vi "Inst.Xeryon-Rotator.GetAllData.vi"(8 "error in (no error)":errorcluster, 11 "Inst.Xeryon-Rotator in":refnum<class "Inst.Xeryon-Rotator.lvclass">) -> (0 "error out":errorcluster, 2 "Data out":variant, 3 "Inst.Xeryon-Rotator out":refnum<class "Inst.Xeryon-Rotator.lvclass">)   [LabVIEW 2019, in "Inst.Xeryon-Rotator.lvclass"]
uses:
  Inst.Xeryon-Rotator.lvclass
  Typedefs/Inst.Xeryon-Rotator.getAll--Cluster.ctl
  Inst.Xeryon-Rotator.lvclass/Inst.Xeryon-Rotator.ctl
  Controller.LV/Controller.LV.lvclass
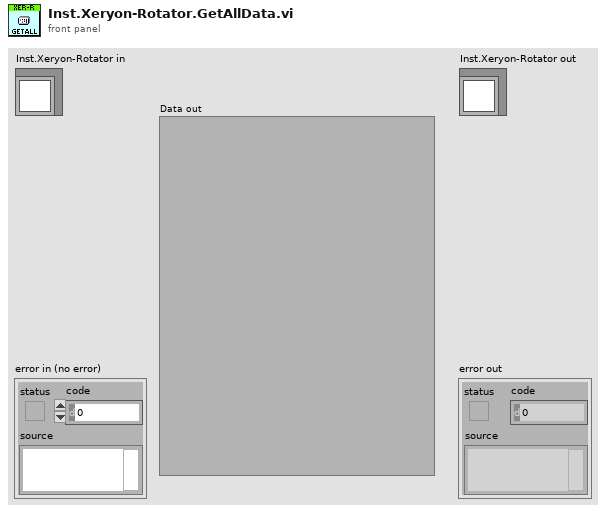
[diagram p1: front panel]
types:
  T1 = typedef "Inst.Xeryon-Rotator.lvclass/Inst.Xeryon-Rotator.getAll--Cluster.ctl" = cluster{"Encoder position [selected units]":dbl, "Desired Position [selected units]":dbl, "Status":string, "SRNO":dbl, "SOFT":dbl, "STAT":dbl, "FREQ":dbl, "OFRQ":dbl, "CURR":dbl, "SYNC":dbl, "Encoder Position [enc. units]":dbl, "Desired Position [enc. units]":dbl, "TIME":dbl, "Index Found":bool, "Left Limit":bool, "Right Limit":bool, "Position Reached":bool}
  T2 = cluster{"SRNO":dbl, "SOFT":dbl, "STAT":dbl, "FREQ":dbl, "OFRQ":dbl, "CURR":dbl, "SYNC":dbl, "Encoder Position [enc. units]":dbl, "Desired Position [enc. units]":dbl, "TIME":dbl}
  T3 = cluster{"Index Found":bool, "Left Limit":bool, "Right Limit":bool, "Position Reached":bool}
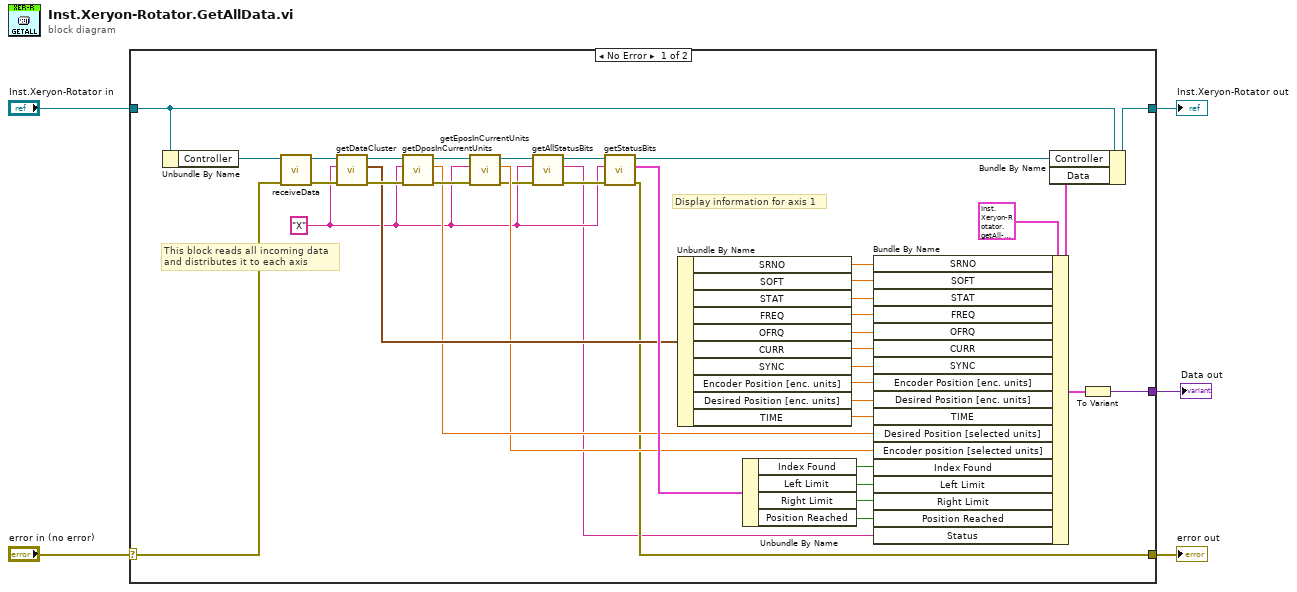
[diagram p0: block diagram]
diagram:
  n1 = case shown="No Error" "error in (no error)" {
    selector: "error in (no error)" -> [w34 w46]
    tunnel: [w13 w46] -> w4
    tunnel: [w44 w45] -> w2
    tunnel: "Inst.Xeryon-Rotator in" -> [w43 w45]
    tunnel: [w42 _] -> w1
    frame No Error {
      w7 = "X" ("Axis Letter")
      # "Display information for axis 1"
      # "This block reads all incoming data\nand distributes it to each axis"
      n2 = Unbundle By Name(w43) -> ("Controller"=w32:refnum<class "Controller.LV.lvclass">)
      n3 = call-dynamic "receiveData.vi"("error in (no error)"=w34, "Controller in"=w32) -> ("error out"=w37:errorcluster, "Controller out"=w36:refnum<class "Controller.LV.lvclass">)  [unwired: 8 in]
      n4 = call-dynamic "getDataCluster.vi"("error in (no error)"=w37, "Axis Letter"=w7, "Controller in"=w36) -> ("error out"=w40:errorcluster, "Information"=w16:T2, "Controller out"=w38:refnum<class "Controller.LV.lvclass">)  [unwired: 6 in]
      n5 = call-dynamic "getDposInCurrentUnits.vi"("error in (no error)"=w40, "Axis Letter"=w7, "Controller in"=w38) -> ("error out"=w41:errorcluster, "DPOS In Current Units"=w15:dbl, "Controller out"=w39:refnum<class "Controller.LV.lvclass">)  [unwired: 6 in]
      n6 = call-dynamic "getEposInCurrentUnits.vi"("error in (no error)"=w41, "Axis Letter"=w7, "Controller in"=w39) -> ("error out"=w10:errorcluster, "EPOS In Current Units"=w14:dbl, "Controller out"=w11:refnum<class "Controller.LV.lvclass">)  [unwired: 6 in]
      n7 = call "getAllStatusBits.vi"("error in (no error)"=w10, "Axis Letter"=w7, "Controller.LV in"=w11) -> ("error out"=w8:errorcluster, "STAT"=w6:string, "Controller.LV out"=w9:refnum<class "Controller.LV.lvclass">)  [unwired: 6 in]
      n8 = call-dynamic "getStatusBits.vi"("error in (no error)"=w8, "Axis Letter"=w7, "Controller in"=w9) -> ("error out"=w13:errorcluster, "StatusBits"=w17:T3, "Controller out"=w35:refnum<class "Controller.LV.lvclass">)  [unwired: 6 in]
      n9 = Unbundle By Name(w16) -> ("SRNO"=w27:dbl, "SOFT"=w26:dbl, "STAT"=w25:dbl, "FREQ"=w24:dbl, "OFRQ"=w23:dbl, "CURR"=w22:dbl, "SYNC"=w21:dbl, "Encoder Position [enc. units]"=w20:dbl, "Desired Position [enc. units]"=w19:dbl, "TIME"=w18:dbl)
      n10 = Unbundle By Name(w17) -> ("Index Found"=w31:bool, "Left Limit"=w30:bool, "Right Limit"=w29:bool, "Position Reached"=w28:bool)
      n11 = Bundle By Name(cluster=T1 {"Encoder position [selected units]"=0.0, "Desired Position [selected units]"=0.0, "Status"="", "SRNO"=0.0, "SOFT"=0.0, "STAT"=0.0, "FREQ"=0.0, "OFRQ"=0.0, "CURR"=0.0, "SYNC"=0.0, "Encoder Position [enc. units]"=0.0, "Desired Position [enc. units]"=0.0, "TIME"=0.0, "Index Found"=FALSE, "Left Limit"=FALSE, "Right Limit"=FALSE, "Position Reached"=FALSE} ("getAll"), "SRNO"=w27, "SOFT"=w26, "STAT"=w25, "FREQ"=w24, "OFRQ"=w23, "CURR"=w22, "SYNC"=w21, "Encoder Position [enc. units]"=w20, "Desired Position [enc. units]"=w19, "TIME"=w18, "Desired Position [selected units]"=w15, "Encoder position [selected units]"=w14, "Index Found"=w31, "Left Limit"=w30, "Right Limit"=w29, "Position Reached"=w28, "Status"=w6) -> (w12:T1)
      n12 = Bundle By Name(cluster=w43, "Controller"=w35, "Data"=w12) -> (w44:refnum<class "Inst.Xeryon-Rotator.lvclass">)
      n13 = To Variant(anything=w12) -> (Variant=w42:variant)
    }
    frame Error {
    }
  }
  "error out" <- w4
  "Inst.Xeryon-Rotator out" <- w2
  "Data out" <- w1
